vi "Utility Number to String.vi"(10 "Numeric":dbl) -> (2 "Shortest String":string)   [LabVIEW 2012, in "Berkeley Nucleonics 500 Series.lvlib"]
doc: "This Utility VI converts a real number to the shortest possible ASCII string. This VI is intended to be used as a private and altering it could cause several public VI's to operate incorrectly."
uses:
  Berkeley Nucleonics 500 Series.lvlib
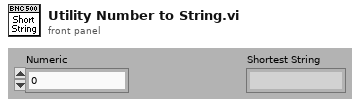
[diagram p1: front panel]
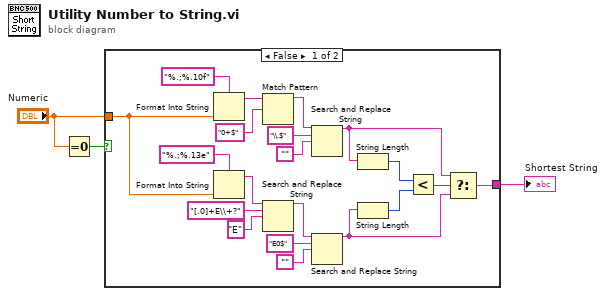
[diagram p0: block diagram]
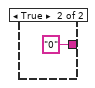
[diagram p2: hidden frame]
diagram:
  n1 = Equal To 0?(x="Numeric") -> (x = 0?=w2:bool)
  n2 = case shown="False" w2 {
    tunnel: [w5 "0" ("result string")] -> w3
    tunnel: "Numeric" -> [w4 _]
    frame False {
      n3 = Format Into String(format string="%.;%.10f", w4) -> (resulting string=w22:string)  [unwired: 2 in, 1 out]
      n4 = Format Into String(format string="%.;%.13e", w4) -> (resulting string=w16:string)  [unwired: 2 in, 1 out]
      n5 = Match Pattern(string=w22, regular expression="0+$") -> (before substring=w11:string)  [unwired: 4 out]
      n6 = Search and Replace String(input string=w16, search string="[.0]+E\\+?", replace string="E" ("replace string (\"\")")) -> (result string=w15:string)  [unwired: 1 in, 7 out]
      n7 = Search and Replace String(input string=w11, search string="\\.$", replace string="" ("replace string (\"\")")) -> (result string=w7:string)  [unwired: 1 in, 7 out]
      n8 = Search and Replace String(input string=w15, search string="E0$", replace string="" ("replace string (\"\")")) -> (result string=w6:string)  [unwired: 1 in, 7 out]
      n9 = String Length(string=w7) -> (length=w10:i32)
      n10 = String Length(string=w6) -> (length=w9:i32)
      n11 = Less?(x=w10, y=w9) -> (x < y?=w8:bool)
      n12 = Select(t=w7, s=w8, f=w6) -> (s? t:f=w5:string)
    }
    frame True {
    }
  }
  "Shortest String" <- w3
